vi "Read.vi"   [LabVIEW 2011, in "Agilent 34401.lvlib"]
doc: "This VI is used to take single, multiple, transient, or math measurements from the multimeter."
uses:
  <instrlib>/Agilent 34401/Agilent 34401.lvlib
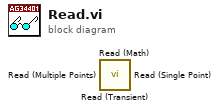
[diagram p0: block diagram]
diagram:
  n1 = call <instrlib>:"Read (Transient).vi"() -> ()  [unwired: 6 in, 6 out]
  n2 = call <instrlib>:"Read (Math).vi"() -> ()  [unwired: 4 in, 8 out]
  n3 = call <instrlib>:"Read (Multiple Points).vi"() -> ()  [unwired: 9 in, 3 out]
  n4 = call <instrlib>:"Read (Single Point).vi"() -> ()  [unwired: 9 in, 3 out]
